vi "ToggleVision.vi"(11 "ButtonArray":bool[](array[boolean])) -> ()   [LabVIEW 2015]
uses:
  VisionGlobals.vi
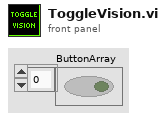
[diagram p1: front panel]
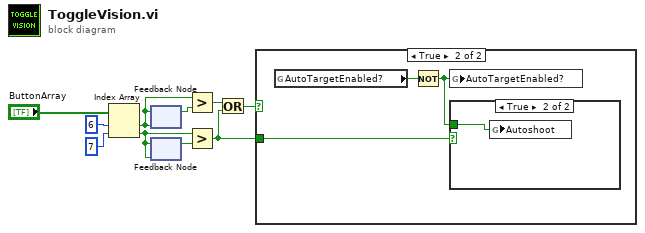
[diagram p0: block diagram]
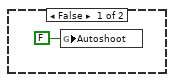
[diagram p3: hidden frame]
diagram:
  n1 = Index Array(array="ButtonArray", index #1=6 ("index"), index #2=7 ("index")) -> (element #1=w8:bool, element #2=w4:bool)
  n2 = feedback-in #1(w8) -> ()
  n3 = feedback #1(w8) -> (w7:bool)
  n4 = feedback #2(w4) -> (w5:bool)
  n5 = feedback-in #2(w4) -> ()
  n6 = Greater?(x=w8, y=w7) -> (0:w2:bool)
  n7 = Greater?(x=w4, y=w5) -> (0:w1:bool)
  n8 = Or(x=w2, y=w1) -> (x .or. y?=w3:bool)
  n9 = case shown="True" w3 {
    tunnel: w1 -> [_ w12]
    frame False {
    }
    frame True {
      n10 = global read "VisionGlobals.vi" "AutoTargetEnabled?"() -> (w13:bool)
      n11 = Not(x=w13) -> (.not. x?=w11:bool)
      n12 = global write "VisionGlobals.vi" "AutoTargetEnabled?"(w11) -> ()
      n13 = case shown="True" w12 {
        tunnel: w11 -> [_ w15]
        frame False {
          n14 = global write "VisionGlobals.vi" "Autoshoot"(FALSE ("Autoshoot")) -> ()
        }
        frame True {
          n15 = global write "VisionGlobals.vi" "Autoshoot"(w15) -> ()
        }
      }
    }
  }
